vi "fit-data-to-range.vi"(1 "in":dbl[](array[numeric])) -> (0 "out":dbl[](array[numeric]))   [LabVIEW 2020]
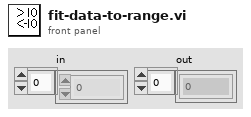
[diagram p1: front panel]
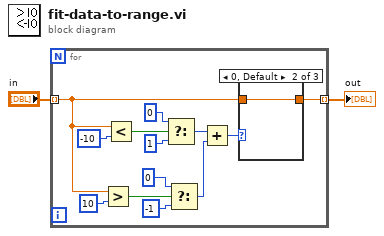
[diagram p0: block diagram]
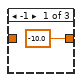
[diagram p2: hidden frame]
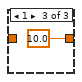
[diagram p3: hidden frame]
diagram:
  n1 = for {
    tunnel: "in" -> [w7] mode=indexing
    tunnel: [w3] -> w1 mode=indexing
    n2 = Greater?(x=w7, y=10) -> (0:w15:bool)
    n3 = Less?(x=w7, y=-10) -> (x < y?=w13:bool)
    n4 = Select(t=0, s=w13, f=1) -> (s? t:f=w12:i32)
    n5 = Select(t=0, s=w15, f=-1) -> (s? t:f=w11:i32)
    n6 = Add(x=w12, y=w11) -> (x+y=w14:i32)
    n7 = case shown="0, Default" w14 {
      tunnel: w7 -> [_ w17 _]
      tunnel: [-10.0 w17 10.0] -> w3
      frame -1 {
      }
      frame 0, Default {
      }
      frame 1 {
      }
    }
  }
  "out" <- w1
